vi "Render Template (Path).vi"(8 "error in (no error)":errorcluster, 10 "Path":path, 11 "Processing in":refnum<class "Processing.lvclass">) -> (0 "error out":errorcluster, 2 "String":string, 3 "Processing out":refnum<class "Processing.lvclass">)   [LabVIEW 2020, in "HTTP Server.lvlib" / "Processing.lvclass"]
uses:
  Processing.lvclass
  Processing.lvclass/Processing.ctl
  TemplateService/TemplateService.lvclass
  C:/dev/lv20CE/relink/lv-http-server/HTTP Server/TemplateService/TemplateService.lvclass
  C:/dev/lv20CE/relink/lv-http-server/HTTP Server/Service/Service.lvclass
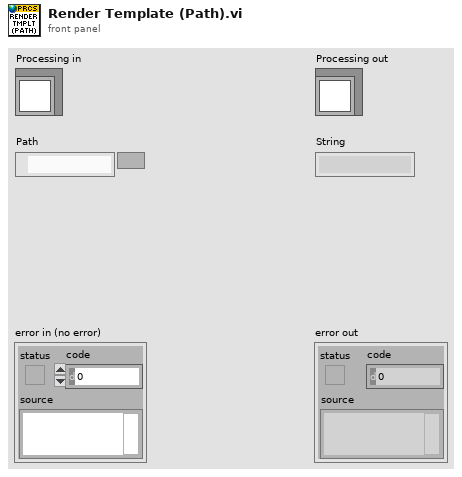
[diagram p1: front panel]
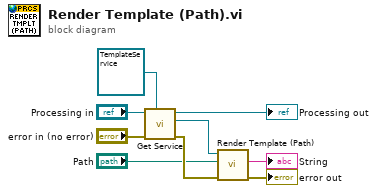
[diagram p0: block diagram]
diagram:
  n1 = call "Get Service.vi"("Service Type"=refnum<class "TemplateService.lvclass"> refnum ("HTTP Server:TemplateService.lvclass"), "error in (no error)"="error in (no error)", "Processing in"="Processing in") -> ("error out"=w7:errorcluster, "Service"=w8:refnum<class "TemplateService.lvclass">, "Processing out"=→"Processing out":refnum<class "Processing.lvclass">)  [unwired: 6 in]
  n2 = call-dynamic "Render Template (Path).vi"("error in (no error)"=w7, "Path"="Path", "TemplateService in"=w8) -> ("error out"=→"error out":errorcluster, "String"=→"String":string)  [unwired: 6 in, 1 out]
